vi "PH_Beamline.set PA DP depending GUI elements.vi"(0 "VI in":refnum<vi>, 5 "error in (no error)":errorcluster) -> (14 "VI out":refnum<vi>, 19 "error out":errorcluster)   [LabVIEW 2014, in "PH_Beamline.lvlib"]
uses:
  PH_Beamline.lvlib
  PH_BL-Master/PH_BL-Master.lvlib
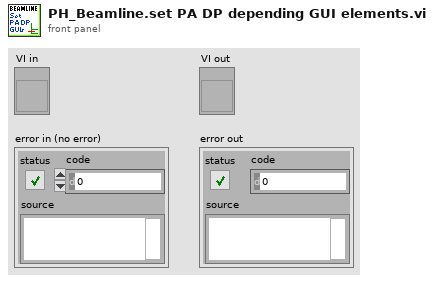
[diagram p1: front panel]
types:
  T1 = typedef "PH_Beamline.lvlib/PH_Beamline.i attribute.ctl" = cluster{"GUI Refs":cluster{"PA ok":refnum<vi>, "MA ok":refnum<vi>, "fs FE ok":refnum<vi>, "ns FE ok":refnum<vi>, "PA ED ok":refnum<vi>, "MAS ok":refnum<vi>, "Booster ok":refnum<vi>, "Mirrortower ok":refnum<vi>, "In.-Box ok":refnum<vi>, "Compressor ok":refnum<vi>, "Experiment LB ok":refnum<vi>, "Experiment LL ok":refnum<vi>, "PHELIX_Beckhoff_Watchdog":refnum<vi>, "Shutters closed":refnum<vi>, "uOPA ok":refnum<vi>, "Vacuum no shotcond Comp LB":refnum<vi>}, "Refs BL MA":refnum<vi>[], "Refs BL MA-IB":refnum<vi>[], "Refs BL fs":refnum<vi>[], "Refs BL PA ED":refnum<vi>[], "Refs BL MAS":refnum<vi>[], "Refs BL Boo":refnum<vi>[], "Refs BL ns":refnum<vi>[], "Refs BL Mirrortower":refnum<vi>[], "Refs BL Compressor":refnum<vi>[], "Refs BL Exp LB":refnum<vi>[], "Radiation Safety":cluster{"Exp Laserbay":cluster{"Ref Op Mode":refnum<vi>, "Ref Laserbay evacuated":refnum<vi>, "Tagname LB evacuated":string, "Shot Mode":T2, "Laserbay evacuated?":i32, "Tagname HV room locked":string, "HV room locked?":i32, "Ref HV room locked":refnum<vi>, "Tagname bridged?":string, "Ref Bridge":refnum<vi>, "I<1E18W/cm²":bool}, "Exp Laserlab":cluster{"Ref Op Mode":refnum<vi>, "Ref Laserlab evacuated":refnum<vi>, "Tagname LL evacuated":string, "Shot Mode":T2, "Laserlab evacuated?":i32, "Tagname bridged?":string, "Ref Bridge":refnum<vi>, "I<1E18W/cm²":bool}}, "Refs BL LL":refnum<vi>[], "PP Igni Heating GUI Refs":refnum<vi>[], "PP Igni Heating Tagnames ":string[], "Refs BL PA":cluster{"undelayed Line before Shutter":refnum<vi>[], "undelayed Line after Shutter":refnum<vi>[], "before Bypass":refnum<vi>[], "delayed Line before Shutter":refnum<vi>[], "delayed Line after Shutter":refnum<vi>[], "before Shutter Input":refnum<vi>[], "after Shutter Input":refnum<vi>[], "Bypass":refnum<vi>[], "before Shutter Exit":refnum<vi>[], "after Shutter Exit":refnum<vi>[], "to MA":refnum<vi>[], "to Lab":refnum<vi>[]}, "BL":cluster{"YLF_BL_Status":i32, "fs_BL_Status":i32, "fs_YLF_BL_Status":i32, "ns_BL_Status":i32, "PA_Input_BL_Status":i32, "PA_UnDelay_BL_Status":i32, "PA_Delay_BL_Status":i32, "PA_BL_Status":i32, "PA_Bypass_BL_Status":i32, "PA_Exit_BL_Status":i32, "PA_LL_BL_Status":i32, "LL_BL_Status":i32, "PA_MA_BL_Status":i32, "MA_Exit_BL_Status":i32, "MA_Z6_BL_Status":i32, "Z6_BL_Status":i32, "MA_LB_BL_Status":i32, "LB_TB2_BL_Status":i32, "PA_before_Bypass_BL_Status":i32, "LB_TB3_BL_Status":i32}, "State Subsystems":cluster{"PA":bool, "MA":bool, "ns FE":bool, "fs FE":bool, "PA ED":bool, "In.-Box":bool, "MAS":bool, "Booster":bool, "Mirrortower":bool, "Compressor":bool, "Experiment LB":bool, "Experiment LL":bool, "uOPA":bool}, "Status Subscriber Information":T3, "Refs BL uOPA":refnum<vi>[], "PA_Input_2_Beam_6PWpGUI not linked?":bool, "PA_Input_Delay_6PGUI not linked?":bool, "Settings":T6}
  T2 = typedef "PH_Beamline.lvlib/PH_Beamline.Operation Mode.ctl" = i32
  T3 = typedef "PH_Beamline.lvlib/PH_Beamline.Status Subscriber Information.ctl" = cluster{"fs Swich YLF":T4, "fs Exit Shutter":T4, "ns Exit Shutter":T4, "PA Input Shutter":T4, "PA PC WP":T4, "PA PC WP 2":T4, "PA Bypass In":T4, "PA Bypass Out":T4, "PA CH 1":T4, "PA delayed":T4, "PA non delayed":T4, "PA Exit Shutter":T4, "PA Switch Lab":T4, "PA Bridge CH Input MA":T4, "MA Diffusor IB":T4, "MA IB Ready":T4, "MA CH 1":T4, "MA CH 2":T4, "MA CH 3":T4, "MA CH 4":T4, "MA Shutter Align Cam":T4, "MA Position MM5":T4, "Calorimeter Switch":T4, "BL Z6 CH 9":T4, "BL Z6 Beamdump":T4, "BL Z6 Shutter":T4, "COS Sensitivity Switch":T4, "Exp LB Shutter":T4, "Exp LB TB 2":T4, "Exp LB TB 3":T4, "PA LL Input CH":T4, "PA LL Output CH":T4, "LL Comp Input Shutter":T4, "LL Comp Output Shutter":T4, "LL Comp FF Shutter":T4, "Exp LL Shutter":T4, "MA IM In IB":T4, "MA IM Out IB":T4, "MA DB In IB":T4, "MA DB Out IB":T4, "Exp LB Shutter Interlock":T4, "Exp LL Shutter Interlock":T4, "MM1 Force Sensor":T4}
  T4 = typedef "PH_BL-Master.lvlib/PH_BL-Master.Status Subscriber Information.ctl" = cluster{"Index of element":i32, "Attributeset":T5}
  T5 = typedef "PH_BL-Master.lvlib/PH_BL-Master.Attribute Set.ctl" = enum16{"Boolean Status Service Subscriber", "Picture Status Service Subscriber"}
  T6 = typedef "PH_Beamline_Chief.lvlib/PH_Beamline_Chief.Settings.ctl" = cluster{"PA Doublepass Mode":bool, "Compressor Vaccuum LB not relevant":bool, "Windowshutter TB2 not relevant":bool, "Windowshutter TB3 not relevant":bool}
  T7 = typedef "PH_BL-Master.lvlib/PH_BL-Master.i attribute.ctl" = cluster{"Remote controlled":bool, "Boolean Condition Service Subscriber":refnum<vi>[], "Picture Condition Service Subscriber":refnum<vi>[], "R2S":cluster{"GUI Ref":refnum<vi>, "State":bool}, "Vacua":cluster{"GUI Ref":refnum<vi>, "Limit":dbl, "Curr Value":dbl, "in range":bool}[], "O2 Inspection":cluster{"GUI Ref":refnum<vi>, "Concentration":dbl, "State":T8}[], "Boolean Status Service Subscriber":cluster{"GUI Ref":refnum<vi>, "Status":T8, "no Link?":bool, "Status Subscriber Class":T9}[], "Picture Status Service Subscriber":cluster{"GUI Ref":refnum<vi>, "Status":T8, "no Link?":bool, "Status Subscriber Class":T9}[], "6P 4Q Service Subscriber":cluster{"GUI Ref":refnum<vi>, "Selector":T10, "no Link?":bool}[], "Index of latest 6P 4Q changing Instance":i32, "Index of latest Picture Status changing Instance":i32, "Index of latest Boolean Status changing Instance":i32, "Vision ID on same Node":string, "Start Phase over?":bool, "GUI Ref Delete":refnum<vi>}
  T8 = typedef "PH_StatusHandler.lvlib/PH_StatusHandler.Status.ctl" = i16
  T9 = typedef "PH_BL-Master.lvlib/PH_BL-Master.Status Subscriber Class.ctl" = enum16{"unknown", "Switch", "BB", "6P Switch", "Switch GUI", "Switch and 6P State", "Force Sensor"}
  T10 = typedef "PH_4_Pos_Selector.lvlib/PH_4_Pos_Selector.Position Selector.ctl" = u16
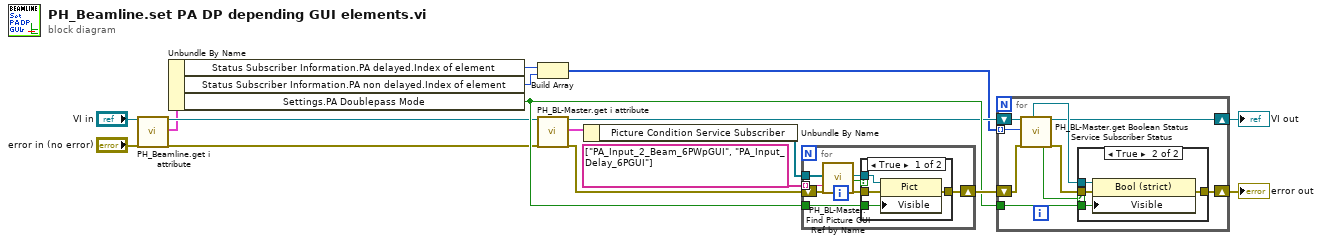
[diagram p0: block diagram]
diagram:
  n1 = call "PH_Beamline.get i attribute.vi"("i ref in"="VI in", "error in (no error)"="error in (no error)") -> ("i ref out"=w10:refnum<vi>, "i attribute"=w2:T1, "error out"=w11:errorcluster)  [unwired: 15 in]
  n2 = Unbundle By Name(w2) -> ("Status Subscriber Information.PA delayed.Index of element"=w3:i32, "Status Subscriber Information.PA non delayed.Index of element"=w4:i32, "Settings.PA Doublepass Mode"=w13:bool)
  n3 = Build Array(w3, w4) -> (w5:i32[])
  n4 = call "PH_BL-Master.get i attribute.vi"("i ref in"=w10, "error in (no error)"=w11) -> ("i ref out"=w12:refnum<vi>, "i attribute"=w8:T7, "error out"=w7:errorcluster)  [unwired: 15 in]
  n5 = Unbundle By Name(w8) -> ("Picture Condition Service Subscriber"=w9:refnum<vi>[])
  n6 = for {
    shift-right: [w21] -> w14
    shift-left: w7 -> [w25]
    tunnel: string[] ["PA_Input_2_Beam_6PWpGUI", "PA_Input_Delay_6PGUI"] -> [w24] mode=indexing
    tunnel: w9 -> [w23]
    tunnel: w13 -> [w18]
    n7 = call "PH_BL-Master.Find Picture GUI Ref by Name.vi"("Pic Ref Array"=w23, "Label"=w24, "error in"=w25) -> ("Wanted Pic GUI Ref"=w20:refnum<vi>, "Ref found?"=w19:bool, "error out"=w22:errorcluster)  [unwired: 13 in, 1 out]
    n8 = case shown="True" w19 {
      tunnel: w22 -> [w29 w30]
      tunnel: [w28 w30] -> w21
      tunnel: w20 -> [w27 _]
      tunnel: w18 -> [w26 _]
      frame True {
        n9 = property class="Pict"(reference=w27, error in=w29, "Visible"=w26) -> (error out=w28:errorcluster)  [unwired: 1 out]
      }
      frame False {
      }
    }
  }
  n10 = for {
    tunnel: w5 -> [w31] mode=indexing
    shift-right: [w37] -> w15
    shift-left: w14 -> [w39]
    tunnel: w13 -> [w35]
    shift-right: [w32] -> w16
    shift-left: w12 -> [w33]
    n11 = call "PH_BL-Master.get Boolean Status Service Subscriber Status.vi"("i ref in"=w33, "Index of wanted element"=w31, "error in (no error)"=w39) -> ("Wanted Boolean Ref"=w36:refnum<vi>, "Information found?"=w34:bool, "i ref out"=w32:refnum<vi>, "error out"=w38:errorcluster)  [unwired: 8 in, 5 out]
    n12 = case shown="True" w34 {
      tunnel: w38 -> [w40 w44]
      tunnel: [w40 w43] -> w37
      tunnel: w36 -> [_ w42]
      tunnel: w35 -> [_ w41]
      frame False {
      }
      frame True {
        n13 = property class="Bool (strict)"(reference=w42, error in=w44, "Visible"=w41) -> (error out=w43:errorcluster)  [unwired: 1 out]
      }
    }
  }
  "VI out" <- w16
  "error out" <- w15
